vi "TableReceiverGoToSkill.vi"(7 "Firstcall?":bool=TRUE, 8 "error in (no error)":errorcluster, 9 "Game":refnum<class "Game.lvclass">, 10 "Robot in":refnum<class "Robot.lvclass">, 11 "TableReceiverGoToSkill in":refnum<class "TableReceiverGoToSkill.lvclass">) -> (0 "error out":errorcluster, 2 "Robot out":refnum<class "Robot.lvclass">, 3 "TableReceiverGoToSkill out":refnum<class "TableReceiverGoToSkill.lvclass">)   [LabVIEW 2018, in "TableReceiverGoToSkill.lvclass"]
uses:
  TableReceiverGoToSkill.lvclass
  Game_class/Game.lvclass
  Robot_class/Robot.lvclass
  Robot_class/roles.ctl
  Game_class/Game.lvclass/Game.ctl
  Object_class/Object.lvclass/Object.ctl
  Parameters_class/Parameters.lvclass/Parameters.ctl
  Team_class/Team.lvclass/Team.ctl
  Robot_class/Robot.lvclass/Robot.ctl
  Object_class/Read x.vi
  Object_class/Read y.vi
  Game_class/Read Utilities.lvclass.vi
  Game_class/Read BallRef.vi
  Game_class/Read FieldRef.vi
  Game_class/Read Parameters.lvclass.vi
  Game_class/Read OffensiveTeam.vi
  Team_class/Read OffensivePlay.vi
  Team_class/Read RobotRef.vi
  Parameters_class/Read AttakingOurselves.vi
  Robot_class/Write dest_x.vi
  Robot_class/Write dest_y.vi
  Robot_class/Write dest_orientation.vi
  Ally_class/Ally.lvclass
  Ball_class/Ball.lvclass
  Utilities_class/Utilities.lvclass
  Field_class/Field.lvclass
  Parameters_class/Parameters.lvclass
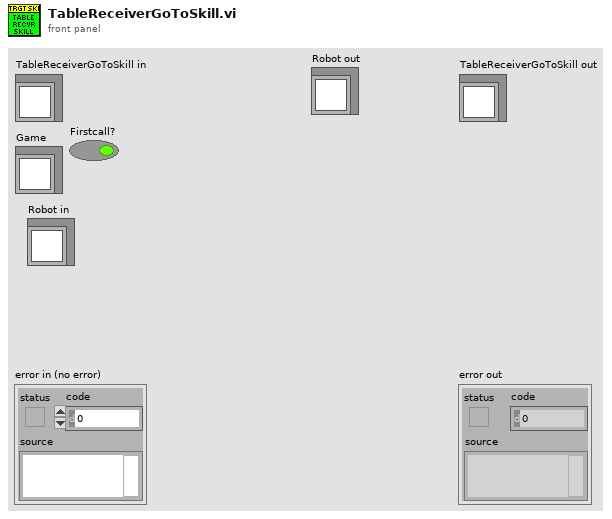
[diagram p1: front panel]
types:
  T1 = typedef "roles.ctl" = enum16{"Tabler", "TableFinalizer", "PrepareRollToPassRoller", "PrepareRollToPassReceiver", "SimplePassRoll", "SimplePassRollReceiver", "PenaltyDefense", "PreparePassReceiver 2", "PreparePassReceiver 1", "PassObserver", "Timeout", "Goto", "ZigZag", "None", "BallOutOfField", "DefenderArea", "Duelist", "AttackerStop", "FollowAttacker", "KeeperRole", "KickPenalty", "AttackerAimGoal", "AttackerBlock", "Marker", "Halt", "Shoot", "PassKicker", "PassReceiver", "TestRole", "PenaltyAttacker"}
  T2 = typedef "OffensivePlay.ctl" = enum16{"TableWithStriker", "TableWith2ndStrikerPlay", "PrepareDoublePass", "PrepareRollToPass", "SimplePass", "PreparePass", "PassToStriker", "BallOutOfField", "PassTo2ndStriker", "StopOffensive", "Prepare Penalty Enemy", "EnemyPossessionAtEnemyField", "EnemyPossesionAtOurField", "TestPlay", "PreparePenaltyAlly", "KickPenaltyAlly", "PrepareKickoffAlly", "PrepareKickoffEnemy", "IndirectEnemy", "DirectEnemy", "NormalGame", "DirectKick", "Pass", "Halt", "Timeout", "PassPlay", "PenaltyEnemy"}
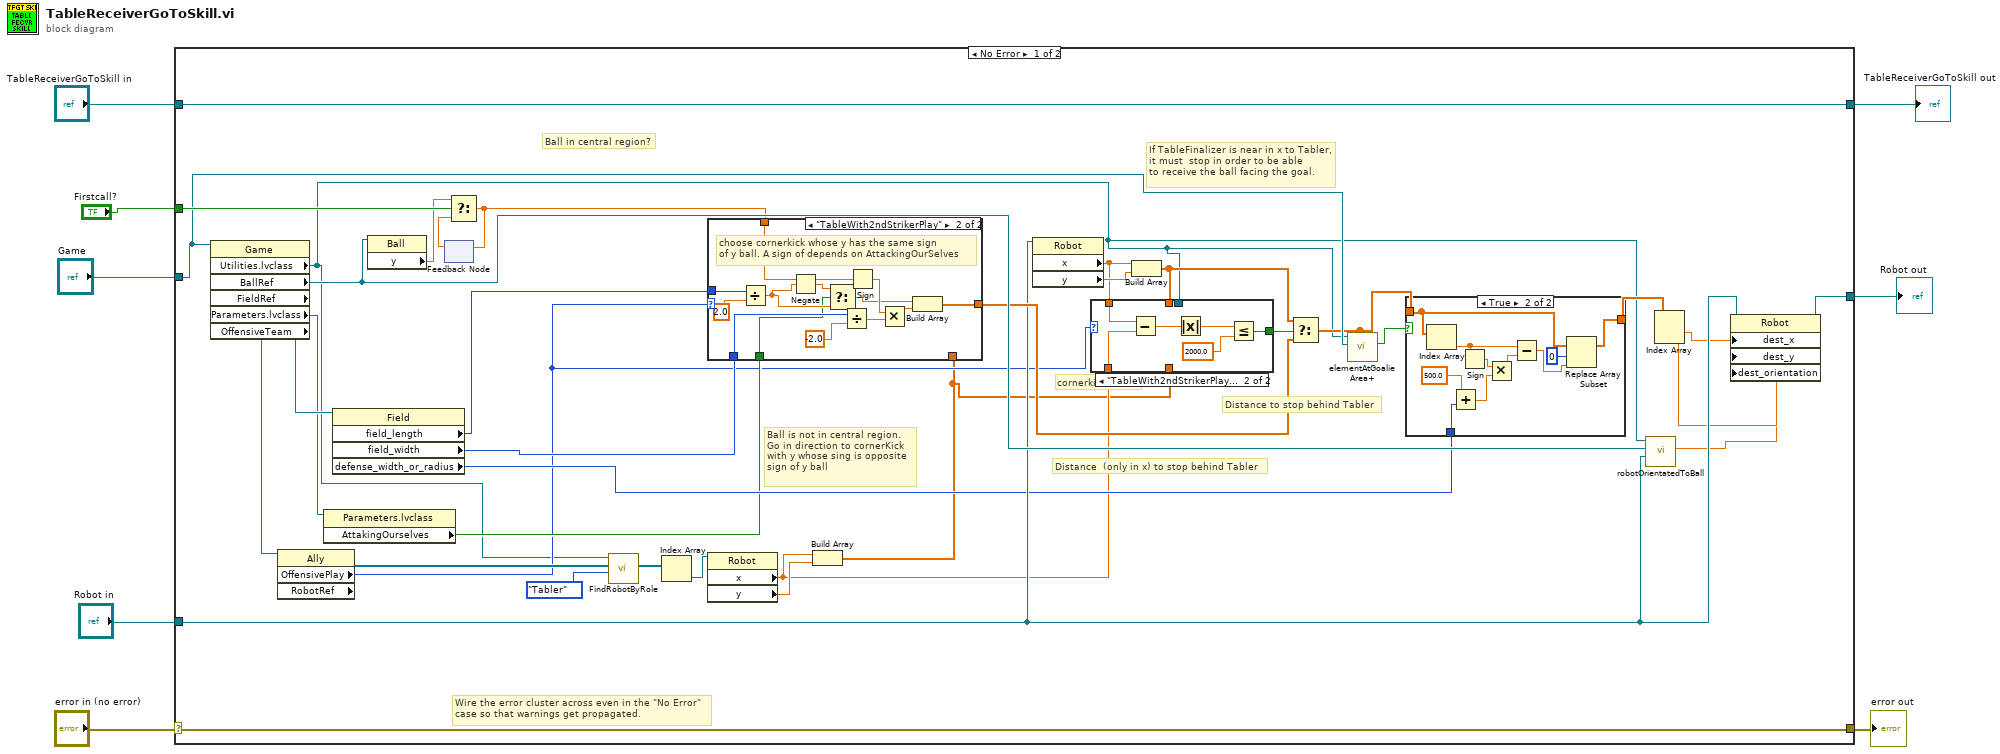
[diagram p0: block diagram]
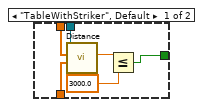
[diagram p2: hidden frame]
diagram:
  n1 = case shown="No Error" "error in (no error)" {
    selector: "error in (no error)" -> [w44 w84]
    tunnel: [w44 w84] -> w7
    tunnel: [w45 w83] -> w5
    tunnel: "TableReceiverGoToSkill in" -> [w45 w83]
    tunnel: "Game" -> [w21 _]
    tunnel: "Robot in" -> [w31 _]
    tunnel: [w27 _] -> w2
    tunnel: "Firstcall?" -> [w26 _]
    frame No Error {
      # "Distance to stop behind Tabler"
      # "cornerkick Point"
      # "Ball is not in central region.\nGo in direction to cornerKick\nwith y whose sing is opposite\nsign of y ball"
      # "Distance  (only in x) to stop behind Tabler"
      # "If TableFinalizer is near in x to Tabler,\nit must  stop in order to be able\nto receive the ball facing the goal."
      # "Ball in central region?"
      # "Wire the error cluster across even in the \"No Error\"\ncase so that warnings get propagated."
      n2 = property class="Game"(reference=w21) -> ("Utilities.lvclass"=w9:refnum<class "Utilities.lvclass">, "BallRef"=w40:refnum<class "Ball.lvclass">, "FieldRef"=w43:refnum<class "Field.lvclass">, "Parameters.lvclass"=w42:refnum<class "Parameters.lvclass">, "OffensiveTeam"=w33:refnum<class "Ally.lvclass">)  [unwired: 1 in, 2 out]
      n3 = property class="Ally"(reference=w33) -> ("OffensivePlay"=w12:T2, "RobotRef"=w32:refnum<class "Robot.lvclass">[])  [unwired: 1 in, 2 out]
      n4 = property class="Parameters.lvclass"(reference=w42) -> ("AttakingOurselves"=w16:bool)  [unwired: 1 in, 2 out]
      n5 = property class="Field"(reference=w43) -> ("field_length"=w15:i32, "field_width"=w41:i32, "defense_width_or_radius"=w18:i32)  [unwired: 1 in, 2 out]
      n6 = property class="Ball"(reference=w40) -> ("y"=w25:dbl)  [unwired: 1 in, 2 out]
      n7 = feedback #1() -> (w24:dbl)  [unwired: 1 in]
      n8 = Select(t=w25, s=w26, f=w24) -> (s? t:f=w23:dbl)
      n9 = feedback-in #1(w23) -> ()
      n10 = call "FindRobotByRole.vi"("role"=roles."Tabler", "RobotRef"=w32, "Utilities in"=w9) -> ("Robots"=w39:refnum<class "Robot.lvclass">[])  [unwired: 6 in, 2 out]
      n11 = Index Array(array=w39) -> (element=w38:refnum<class "Robot.lvclass">)  [unwired: 1 in]
      n12 = property class="Robot"(reference=w38) -> ("x"=w13:dbl, "y"=w14:dbl)  [unwired: 1 in, 2 out]
      n13 = Build Array(w13, w14) -> (w10:dbl[])
      n14 = case shown="\"TableWith2ndStrikerPlay\"" w12 {
        tunnel: w41 -> [_ w71]
        tunnel: [w58 w70] -> w36
        tunnel: w23 -> [_ w69]
        tunnel: w16 -> [_ w62]
        tunnel: w15 -> [_ w61]
        tunnel: w10 -> [w58 _]
        frame "TableWithStriker", Default {
          # "Go in direction to Tabler"
        }
        frame "TableWith2ndStrikerPlay" {
          # "choose cornerkick whose y has the same sign\nof y ball. A sign of depends on AttackingOurSelves"
          n15 = Divide(x=w61, y=2.0) -> (x/y=w63:dbl)
          n16 = Negate(x=w63) -> (-x=w64:dbl)
          n17 = Select(t=w64, s=w62, f=w63) -> (s? t:f=w60:dbl)
          n18 = Divide(x=w71, y=-2.0) -> (x/y=w66:dbl)
          n19 = Sign(1:w69) -> (0:w67:dbl)
          n20 = Multiply(x=w67, y=w66) -> (x*y=w68:dbl)
          n21 = Build Array(w60, w68) -> (w70:dbl[])
        }
      }
      n22 = property class="Robot"(reference=w31) -> ("x"=w22:dbl, "y"=w35:dbl)  [unwired: 1 in, 2 out]
      n23 = Build Array(w22, w35) -> (w11:dbl[])
      n24 = case shown="\"TableWith2ndStrikerPlay\"" w12 {
        tunnel: [w50 w55] -> w37
        tunnel: w22 -> [_ w54]
        tunnel: w13 -> [_ w53]
        tunnel: w11 -> [w48 _]
        tunnel: w10 -> [w49 _]
        tunnel: w9 -> [w47 _]
        frame "TableWithStriker", Default {
          n25 = call-dynamic "Distance.vi"("P1"=w49, "P2"=w48, "Utilities in"=w47) -> ("Distance"=w51:dbl)  [unwired: 6 in, 2 out]
          n26 = Less Or Equal?(x=w51, y=3000.0) -> (x <= y?=w50:bool)
        }
        frame "TableWith2ndStrikerPlay" {
          n27 = Subtract(x=w54, y=w53) -> (x-y=w57:dbl)
          n28 = Absolute Value(x=w57) -> (abs(x)=w56:dbl)
          n29 = Less Or Equal?(x=w56, y=2000.0) -> (x <= y?=w55:bool)
        }
      }
      n30 = Select(t=w11, s=w37, f=w36) -> (s? t:f=w17:dbl[])
      n31 = call "elementAtGoalieArea+.vi"("Elemento pos."=w17, "Game"=w21, "Utilities in"=w9) -> ("Elemento at goalkeeper area + ?"=w20:bool)  [unwired: 6 in, 2 out]
      n32 = case shown="True" w20 {
        tunnel: w17 -> [w72 w81]
        tunnel: [w72 w79] -> w19
        tunnel: w18 -> [_ w73]
        frame False {
        }
        frame True {
          n33 = Index Array(array=w81) -> (element=w78:dbl)  [unwired: 1 in]
          n34 = Add(x=500.0, y=w73) -> (x+y=w75:dbl)
          n35 = Sign(1:w78) -> (0:w80:dbl)
          n36 = Multiply(x=w80, y=w75) -> (x*y=w77:dbl)
          n37 = Subtract(x=w78, y=w77) -> (x-y=w76:dbl)
          n38 = Replace Array Subset(array=w81, new element=w76, index=0) -> (w79:dbl[])
        }
      }
      n39 = call "robotOrientatedToBall.vi"("Robot"=w31, "BallRef"=w40, "Utilities in"=w9) -> ("Orientation"=w28:dbl)  [unwired: 6 in, 2 out]
      n40 = Index Array(array=w19) -> (element #1=w30:dbl, element #2=w29:dbl)  [unwired: 2 in]
      n41 = property class="Robot"(reference=w31, "dest_x"=w30, "dest_y"=w29, "dest_orientation"=w28) -> (reference out=w27:refnum<class "Robot.lvclass">)  [unwired: 1 in, 1 out]
    }
    frame Error {
    }
  }
  "error out" <- w7
  "TableReceiverGoToSkill out" <- w5
  "Robot out" <- w2
